vi "Add AQT to Tree.vi"(9 "Current AQT List":string[](array[string]), 10 "AQT Name":string, 11 "TreeControl in":refnum<vi>) -> (0 "error out":errorcluster)   [LabVIEW 2025]
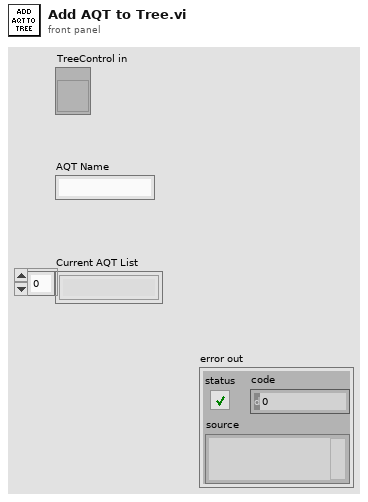
[diagram p1: front panel]
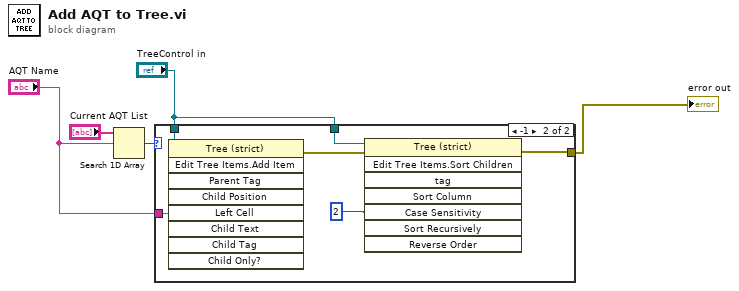
[diagram p0: block diagram]
diagram:
  n1 = Search 1D Array(1D array="Current AQT List", element="AQT Name") -> (index of element=w2:i32)  [unwired: 1 in]
  n2 = case shown="-1" w2 {
    tunnel: [_ w8] -> w4
    tunnel: "AQT Name" -> [_ w11]
    tunnel: "TreeControl in" -> [_ w7]
    tunnel: "TreeControl in" -> [_ w6]
    frame 0, Default {
    }
    frame -1 {
      n3 = invoke on="Invoke Node" class="Tree (strict)" method="Edit Tree Items.Add Item"(reference=w7, "Left Cell"=w11) -> (error out=w9:errorcluster)  [unwired: 7 in, 8 out]
      n4 = invoke on="Invoke Node" class="Tree (strict)" method="Edit Tree Items.Sort Children"(reference=w6, error in=w9, "Case Sensitivity"=2) -> (error out=w8:errorcluster)  [unwired: 5 in, 7 out]
    }
  }
  "error out" <- w4
